vi "SRV_TCP Read Data.vi"(4 "TCP Settings":T1={"Method"=enum."General", "bytes to read"=2000, "timeout ms (1000)"=1000}, 5 "error in":errorcluster, 8 "connection ID in":refnum<k5>) -> (0 "error out":errorcluster, 1 "data out":string, 3 "connection ID":refnum<k5>, 6 "Size read":i32)   [LabVIEW 2014]
doc: "Read information from the SRV.\n\n\nModified for Benilde St. Margaret's School - Tim Jump\nBy Doug Schmertman - Logic PD\nCopyright 2012"
uses:
  SRV_TCP Settings.ctl
  SRV_Package Methods.ctl
panel:
  out "Image size":i32
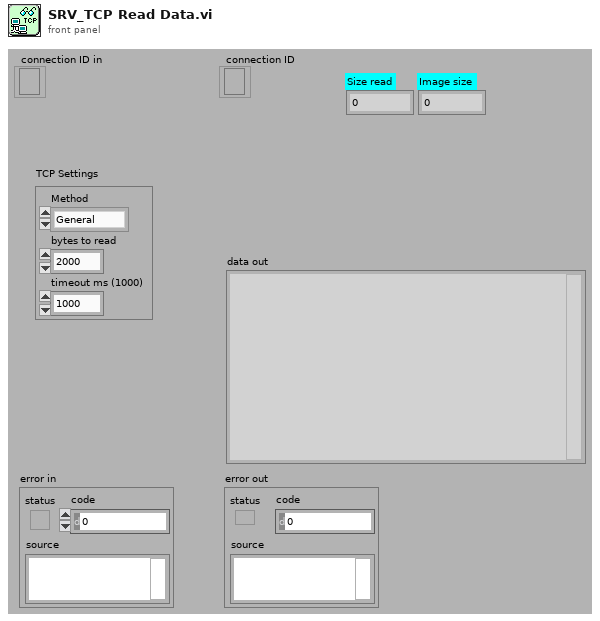
[diagram p1: front panel]
types:
  T1 = typedef "SRV_TCP Settings.ctl" = cluster{"Method":T2, "bytes to read":i32, "timeout ms (1000)":i32}
  T2 = typedef "SRV_Package Methods.ctl" = enum16{"General", "Standard", "CRLF", "Image", "HTML"}
  T3 = enum16{"Standard", "Buffered", "CRLF", "Immediate"}
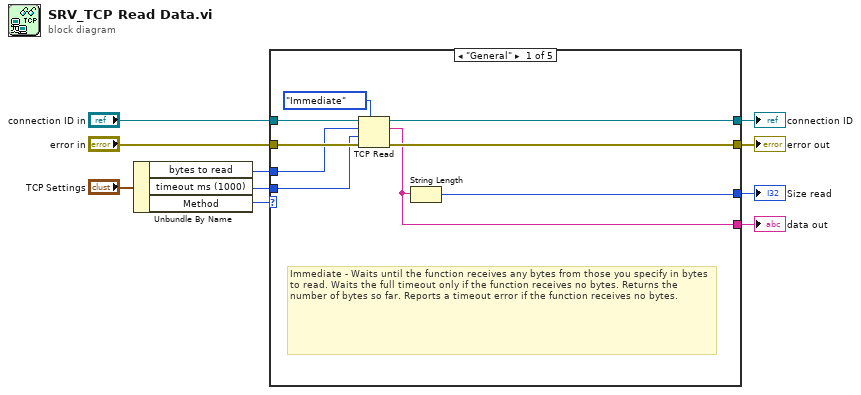
[diagram p0: block diagram]
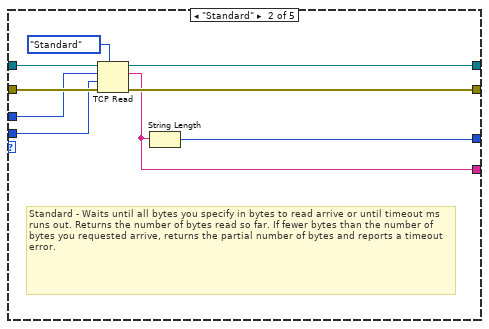
[diagram p2: hidden frame]
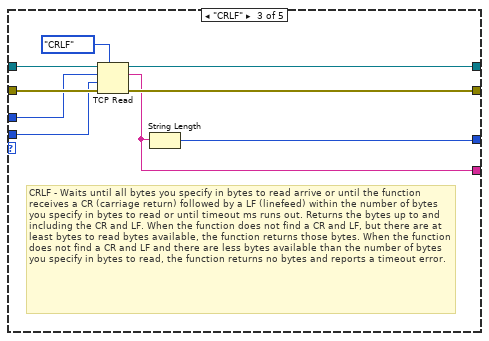
[diagram p3: hidden frame]
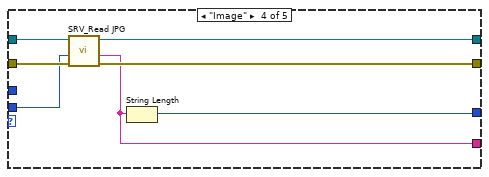
[diagram p4: hidden frame]
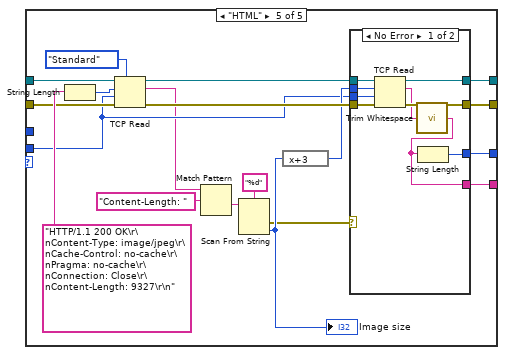
[diagram p5: hidden frame]
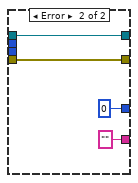
[diagram p6: hidden frame]
diagram:
  n1 = Unbundle By Name("TCP Settings") -> ("bytes to read"=w2:i32, "timeout ms (1000)"=w3:i32, "Method"=w1:T2)
  n2 = case shown="\"General\"" w1 {
    tunnel: [w15 w24 w33 w41 w61] -> w10
    tunnel: [w13 w22 w29 w39 w60] -> w9
    tunnel: [w16 w25 w34 w40 w56] -> w8
    tunnel: [w14 w23 w32 w42 w55] -> w4
    tunnel: "connection ID in" -> [w19 w28 w37 w44 w50]
    tunnel: "error in" -> [w18 w27 w36 w43 w49]
    tunnel: w3 -> [w12 w21 w31 w38 w46]
    tunnel: w2 -> [w11 w20 w30 _ _]
    frame "General" {
      # "Immediate - Waits until the function receives any bytes from those you specify in bytes to read. Waits the full timeout only if the function receives no bytes. Returns the number of bytes so far. Reports a timeout error if the function receives no bytes."
      n3 = TCP Read(connection ID=w19, bytes to read=w11, error in (no error)=w18, 7:T3."Immediate" ("mode (standard)"), 9:w12) -> (connection ID out=w14:refnum<k5>, data out=w13:string, error out=w15:errorcluster)
      n4 = String Length(string=w13) -> (length=w16:i32)
    }
    frame "Standard" {
      # "Standard - Waits until all bytes you specify in bytes to read arrive or until timeout ms runs out. Returns the number of bytes read so far. If fewer bytes than the number of bytes you requested arrive, returns the partial number of bytes and reports a timeout error."
      n5 = TCP Read(connection ID=w28, bytes to read=w20, error in (no error)=w27, 7:T3."Standard" ("mode (standard)"), 9:w21) -> (connection ID out=w23:refnum<k5>, data out=w22:string, error out=w24:errorcluster)
      n6 = String Length(string=w22) -> (length=w25:i32)
    }
    frame "CRLF" {
      # "CRLF - Waits until all bytes you specify in bytes to read arrive or until the function receives a CR (carriage return) followed by a LF (linefeed) within the number of bytes you specify in bytes to read or until timeout ms runs out. Returns the bytes up to and including the CR and LF. When the function does not find a CR and LF, but there are at least bytes to read bytes available, the function returns those bytes. When the function does not find a CR and LF and there are less bytes available than the number of bytes you specify in bytes to read, the function returns no bytes and reports a timeout error."
      n7 = TCP Read(connection ID=w37, bytes to read=w30, error in (no error)=w36, 7:T3."CRLF" ("mode (standard)"), 9:w31) -> (connection ID out=w32:refnum<k5>, data out=w29:string, error out=w33:errorcluster)
      n8 = String Length(string=w29) -> (length=w34:i32)
    }
    frame "Image" {
      n9 = call "SRV_Read JPG.vi"("error in"=w43, "timeout ms (25000)"=w38, "connection ID in"=w44) -> ("error out"=w41:errorcluster, "data out"=w39:string, "connection ID"=w42:refnum<k5>)  [unwired: 6 in]
      n10 = String Length(string=w39) -> (length=w40:i32)
    }
    frame "HTML" {
      n11 = String Length(string="HTTP/1.1 200 OK\r\nContent-Type: image/jpeg\r\nCache-Control: no-cache\r\nPragma: no-cache\r\nConnection: Close\r\nContent-Length: 9327\r\n" ("IP address 2")) -> (length=w63:i32)
      n12 = TCP Read(connection ID=w50, bytes to read=w63, error in (no error)=w49, 7:T3."Standard" ("mode (standard)"), 9:w46) -> (connection ID out=w54:refnum<k5>, data out=w45:string, error out=w59:errorcluster)
      n13 = Match Pattern(string=w45, regular expression="Content-Length: ") -> (after substring=w52:string)  [unwired: 1 in, 3 out]
      n14 = Scan From String(format string="%d", input string=w52) -> (error out=w47:errorcluster, output 1=w57:i32)  [unwired: 3 in, 2 out]
      "Image size" <- w57
      n15 = expression code="x+3"(w57) -> (w58:i32)
      n16 = case shown="No Error" w47 {
        tunnel: [w72 w75] -> w61
        tunnel: [w64 "" ("trimmed string")] -> w60
        tunnel: w59 -> [w71 w75]
        tunnel: w58 -> [w70 _]
        tunnel: [w69 0] -> w56
        tunnel: w46 -> [w67 _]
        tunnel: [w66 w76] -> w55
        tunnel: w54 -> [w65 w76]
        frame No Error {
          n17 = TCP Read(connection ID=w65, bytes to read=w70, error in (no error)=w71, 9:w67) -> (connection ID out=w66:refnum<k5>, data out=w68:string, error out=w72:errorcluster)  [unwired: 1 in]
          n18 = call <vilib>:"Trim Whitespace.vi"("string"=w68) -> ("trimmed string"=w64:string)  [unwired: 1 in]
          n19 = String Length(string=w64) -> (length=w69:i32)
        }
        frame Error {
        }
      }
    }
  }
  "data out" <- w9
  "Size read" <- w8
  "error out" <- w10
  "connection ID" <- w4
